vi "Drive Capacity GB.vi"(8 "error in (no error)":errorcluster, 10 "Path":path, 11 "Windows System SAL in":refnum<class "Windows System SAL.lvclass">) -> (0 "error out":errorcluster, 2 "Capacity GB":dbl, 3 "Windows System SAL out":refnum<class "Windows System SAL.lvclass">)   [LabVIEW 2020, in "Volatus.lvlib" / "Windows System SAL.lvclass"]
uses:
  Windows System SAL.lvclass
  Windows System SAL.lvclass/Windows System SAL.ctl
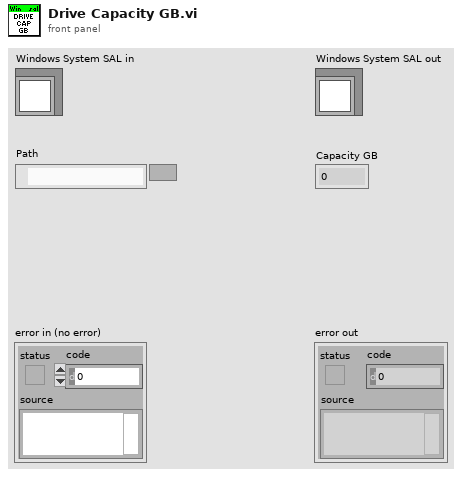
[diagram p1: front panel]
types:
  T1 = typedef "Volatus.lvlib/Windows System SAL.lvclass/Drive Info.ctl" = cluster{"Size GB":dbl, "Free GB":dbl}
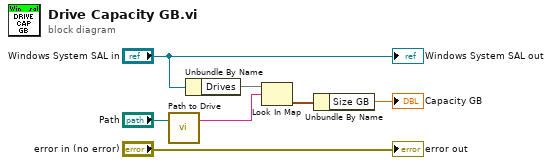
[diagram p0: block diagram]
diagram:
  n1 = call "Path to Drive.vi"("Path"="Path") -> ("Drive"=w3:string)  [unwired: 6 in]
  n2 = Unbundle By Name("Windows System SAL in") -> ("Drives"=w4:map{string, T1})
  n3 = Look In Map(map=w4, key=w3) -> (value=w2:T1)  [unwired: 1 in, 1 out]
  n4 = Unbundle By Name(w2) -> ("Size GB"=→"Capacity GB":dbl)
  "error out" <- "error in (no error)"
  "Windows System SAL out" <- "Windows System SAL in"
